vi "特殊方法创建的枚举控件.vi"() -> ()   [LabVIEW 2012]
panel:
  in  "枚举 2":enum16{"≠", "＝", "＞", "≥", "＜", "≤"}(ring)
  in  "枚举":enum16{"≠", "＝", "＞", "≥", "＜", "≤"}(ring)
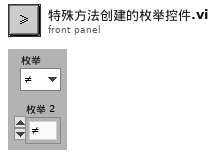
[diagram p1: front panel]
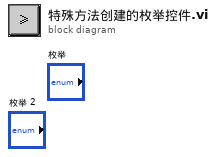
[diagram p0: block diagram]
diagram:
